vi "WaitForPubSetup.vi"(3 "ROS in":T1) -> (1 "ROS out":T1)   [LabVIEW 2012]
doc: "Waits for publisher to start"
uses:
  _ROSDirection.ctl
  _ROSControl.ctl
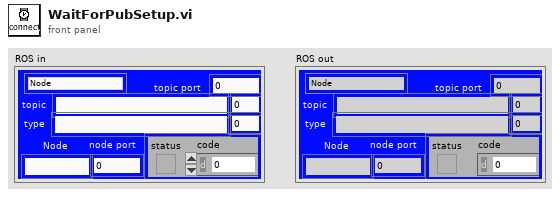
[diagram p1: front panel]
types:
  T1 = typedef "_ROSControl.ctl" = cluster{"topic port":u16, "Node":string, "topic":string, "type":string, "node port":u16, "error ":errorcluster, "Direction":T2, "Update (ms)":u16, "FIFO size":u16}
  T2 = typedef "_ROSDirection.ctl" = enum16{"Node", "Publisher", "Subscriber", "ServiceClient", "ServiceProvider"}
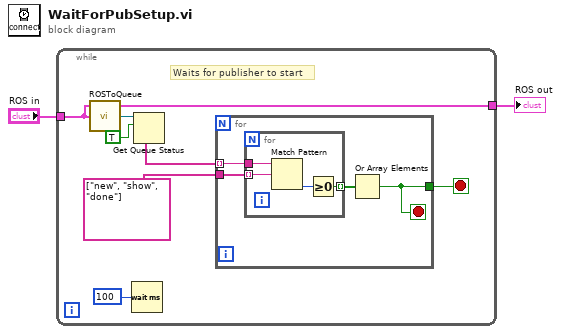
[diagram p0: block diagram]
diagram:
  n1 = while {
    tunnel: "ROS in" -> [w4]
    tunnel: [w4] -> w2
    stop <- w7 stop-if-true
    # "Waits for publisher to start"
    n2 = call "ROSToQueue.vi"("ROS"=w4) -> ("queue"=w9:refnum<queue>)  [unwired: 3 in, 1 out]
    n3 = Wait (ms)(milliseconds to wait=u32 100) -> ()  [unwired: 1 out]
    n4 = Get Queue Status(queue=w9, return elements? (F)=TRUE) -> (elements=w8:string[])  [unwired: 1 in, 7 out]
    n5 = for {
      tunnel: w8 -> [w13] mode=indexing
      tunnel: [w10] -> w7
      tunnel: string[] ["new", "show", "done"] -> [w11]
      stop <- w10 stop-if-true
      n6 = for {
        tunnel: w13 -> [w17]
        tunnel: [w15] -> w12 mode=indexing
        tunnel: w11 -> [w14] mode=indexing
        n7 = Match Pattern(string=w17, regular expression=w14) -> (offset past match=w16:i32)  [unwired: 1 in, 3 out]
        n8 = Greater Or Equal To 0?(x=w16) -> (x >= 0?=w15:bool)
      }
      n9 = Or Array Elements(Boolean array=w12) -> (logical OR=w10:bool)
    }
  }
  "ROS out" <- w2
